vi "Set module data.vi"(8 "error in (no error)":errorcluster, 10 "Position":dbl, 11 "Module in":refnum<class "Module.lvclass">) -> (0 "error out":errorcluster, 3 "Module out":refnum<class "Module.lvclass">)   [LabVIEW 2021, in "Module.lvclass"]
uses:
  Module.lvclass
  Module.lvclass/Module.ctl
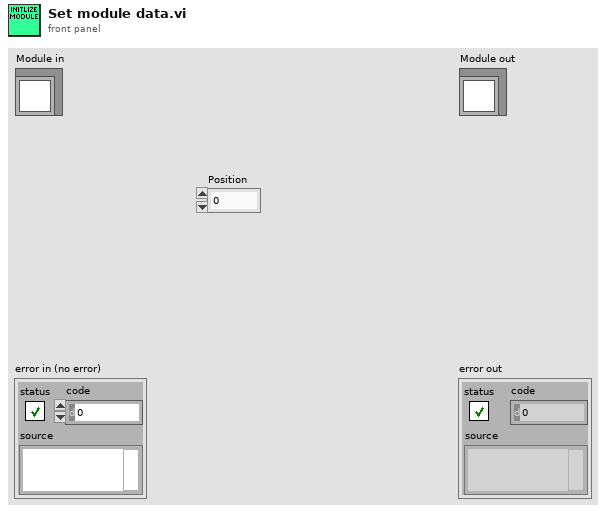
[diagram p1: front panel]
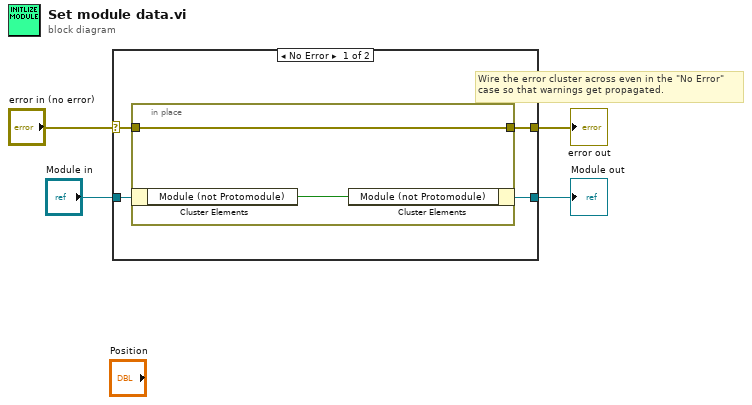
[diagram p0: block diagram]
diagram:
  n1 = case shown="No Error" "error in (no error)" {
    selector: "error in (no error)" -> [w7 w12]
    tunnel: [w6 w12] -> w3
    tunnel: [w5 w11] -> w1
    tunnel: "Module in" -> [w8 w11]
    frame No Error {
      # "Wire the error cluster across even in the \"No Error\"\ncase so that warnings get propagated."
      n2 = in-place {
        in-place-border: w7 -> [w9]
        in-place-border: [w9] -> w6
        n3 = in-place-cluster #1(w8) -> ("Module (not Protomodule)"=w10:bool)
        n4 = in-place-cluster #1("Module (not Protomodule)"=w10) -> (w5:refnum<class "Module.lvclass">)
      }
    }
    frame Error {
    }
  }
  "error out" <- w3
  "Module out" <- w1
